vi "Move XYZA.vi"(3 "Make Vertical":bool=TRUE, 4 "Side":T1=enum."right", 5 "Label":string, 6 "Wait Time":dbl, 8 "error in":errorcluster, 9 "Speed (mm/s)":dbl=50.0, 10 "XYZA":cluster{"X":dbl, "Y":dbl, "Z":dbl, "A":dbl}, 11 "Location":string="Current") -> (0 "error out":errorcluster)   [LabVIEW 2013]
uses:
  ROS/Code/SubVIs/BaxterSide.ctl
  Move XYZOAT.vi
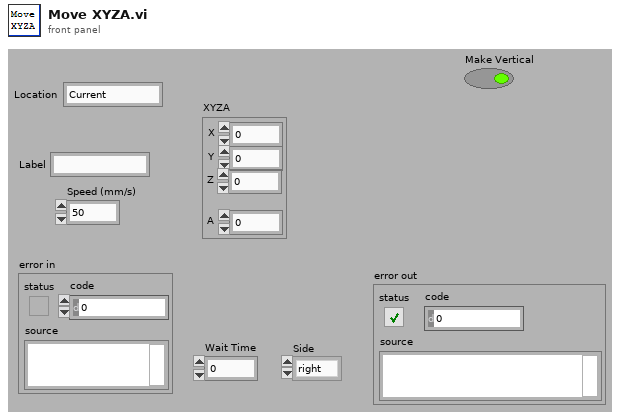
[diagram p1: front panel]
types:
  T1 = typedef "BaxterSide.ctl" = enum16{"left", "right"}
  T2 = cluster{"X":dbl, "Y":dbl, "Z":dbl, "Roll":dbl, "Pitch":dbl, "Yaw":dbl}
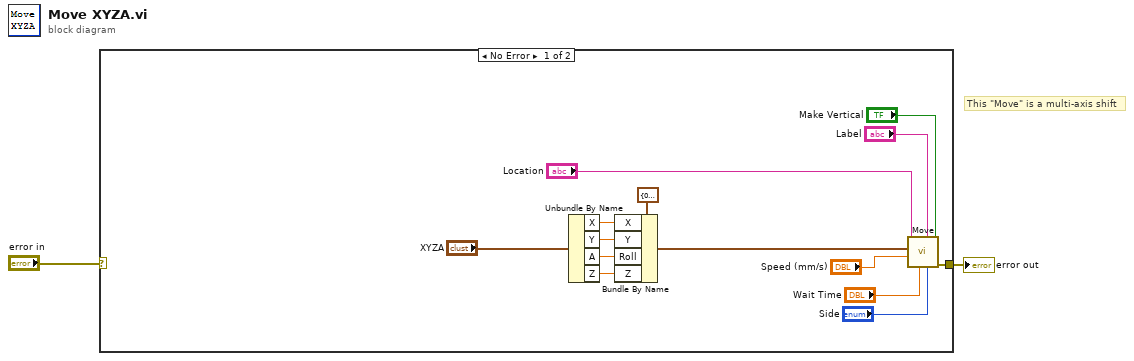
[diagram p0: block diagram]
diagram:
  # "This \"Move\" is a multi-axis shift"
  n1 = case shown="No Error" "error in" {
    selector: "error in" -> [_ w17]
    tunnel: [w15 w17] -> w1
    frame No Error {
      n2 = Unbundle By Name("XYZA") -> ("X"=w6:dbl, "Y"=w7:dbl, "A"=w8:dbl, "Z"=w5:dbl)
      n3 = Bundle By Name(cluster=T2 {"X"=0.0, "Y"=0.0, "Z"=0.0, "Roll"=0.0, "Pitch"=0.0, "Yaw"=0.0} ("XYZOAT"), "X"=w6, "Y"=w7, "Roll"=w8, "Z"=w5) -> (w11:T2)
      n4 = call-poly "Move.vi"("Make Vertical"="Make Vertical", "Side"="Side", "Label"="Label", "Wait Time"="Wait Time", "Speed (mm/s)"="Speed (mm/s)", "XYZOAT"=w11, "Location"="Location") -> ("error out"=w15:errorcluster)  [unwired: 4 in]
    }
    frame Error {
    }
  }
  "error out" <- w1
